vi "Check mtcdt check wifi scan.vi"(6 "VISA resource name":refnum<visa-resource-name>="COM5", 7 "Passed so far":bool, 8 "error in (no error)":errorcluster) -> (0 "error out":errorcluster, 3 "wifi mac":string, 4 "VISA Refnum out":refnum<visa-resource-name>, 5 "Passed?":bool)   [LabVIEW 2024]
panel:
  out "Response 6":string
  out "response":string
  out "Response 5":string
  out "Response 4":string
  out "Response 3":string
  out "Response 2":string
  out "Response":string
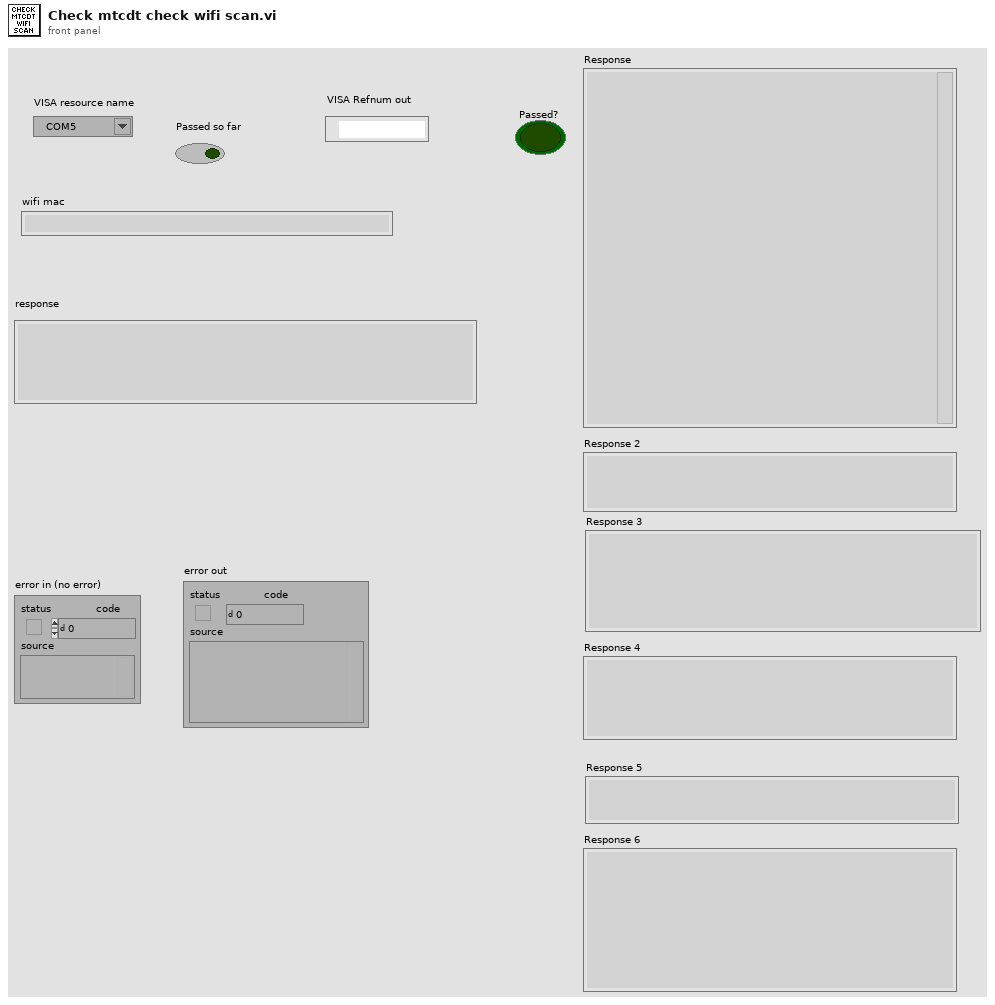
[diagram p1: front panel]
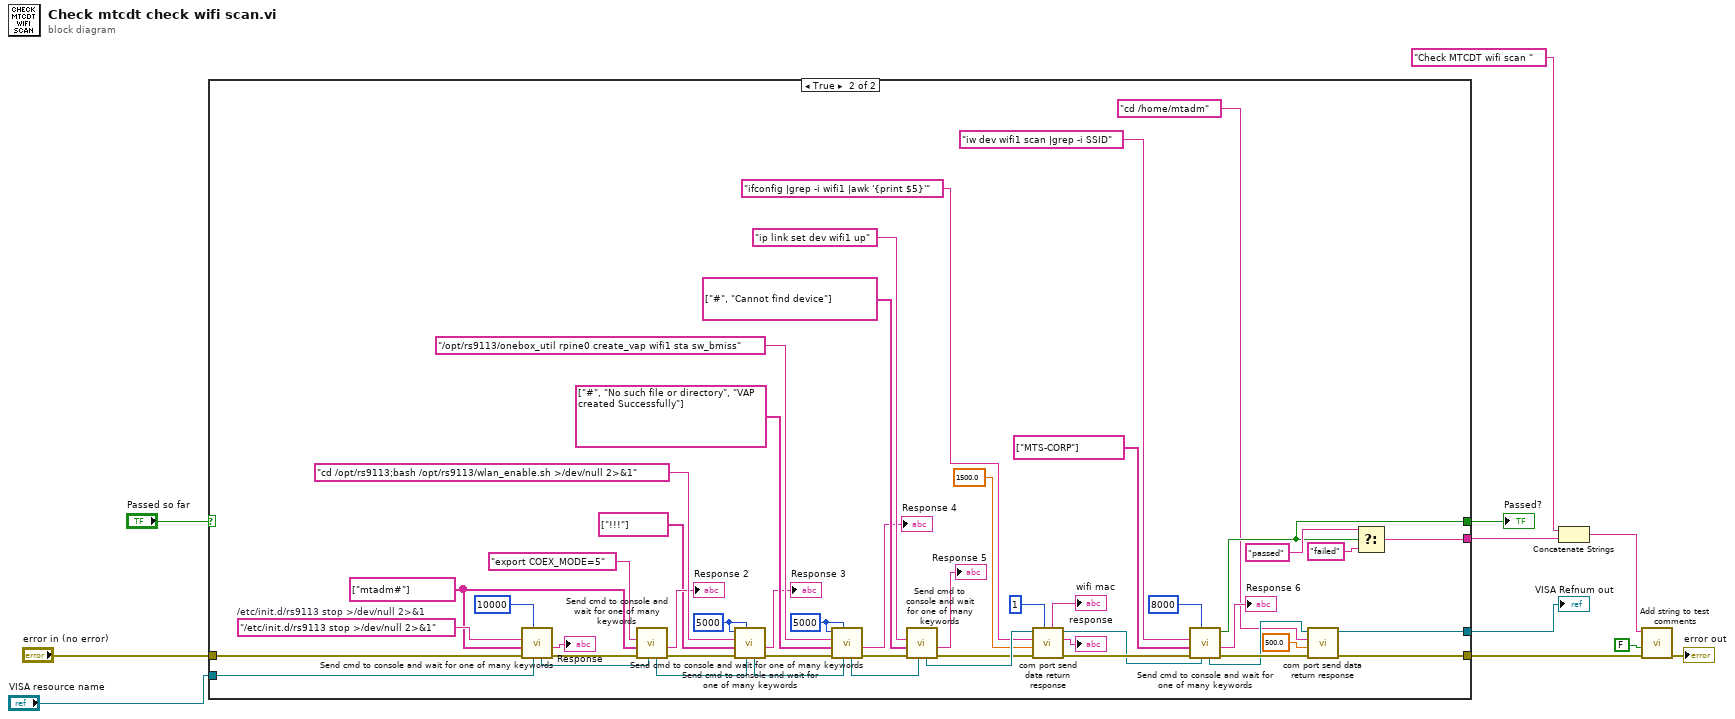
[diagram p0: block diagram]
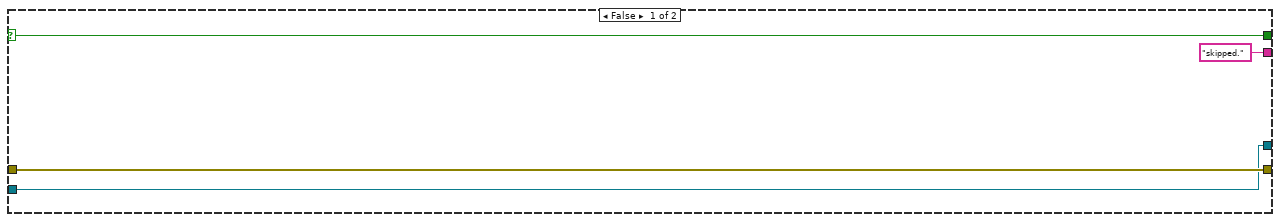
[diagram p2: hidden frame]
diagram:
  n1 = case shown="True" "Passed so far" {
    selector: "Passed so far" -> [w15 _]
    tunnel: "error in (no error)" -> [w14 w65]
    tunnel: [w14 w20] -> w2
    tunnel: "VISA resource name" -> [w13 w64]
    tunnel: [w15 w23] -> w6
    tunnel: [w13 w18] -> w4
    tunnel: ["skipped." w22] -> w1
    frame False {
    }
    frame True {
      w26 = u32 5000 ("Wait after send")
      w27 = u32 5000 ("Timeout (1000 mSecs)")
      w59 = string[] ["mtadm#"] ("Wait for keywords")
      w63 = "/etc/init.d/rs9113 stop >/dev/null 2>&1"  # /etc/init.d/rs9113 stop >/dev/null 2>&1
      n2 = call "Send cmd to console and wait for one of many keywords.vi"("VISA resource name"=w64, "Timeout (1000 mSecs)"=u32 10000, "error in (no error)"=w65, "Wait for keywords"=w59, "cmd"=w63) -> ("error out"=w60:errorcluster, "Response"=→"Response":string, "VISA Refnum out"=w62:refnum<visa-resource-name>)  [unwired: 2 in, 2 out]
      n3 = call "Send cmd to console and wait for one of many keywords.vi"("VISA resource name"=w62, "error in (no error)"=w60, "Wait for keywords"=w59, "cmd"="export COEX_MODE=5" ("write buffer")) -> ("error out"=w57:errorcluster, "Response"=→"Response 2":string, "VISA Refnum out"=w56:refnum<visa-resource-name>)  [unwired: 3 in, 2 out]
      n4 = call "Send cmd to console and wait for one of many keywords.vi"("VISA resource name"=w56, "Timeout (1000 mSecs)"=w26, "error in (no error)"=w57, "Wait for keywords"=string[] ["!!!"], "cmd"="cd /opt/rs9113;bash /opt/rs9113/wlan_enable.sh >/dev/null 2>&1" ("write buffer"), "Wait after send"=w26) -> ("error out"=w53:errorcluster, "Response"=→"Response 3":string, "VISA Refnum out"=w52:refnum<visa-resource-name>)  [unwired: 1 in, 2 out]
      n5 = call "Send cmd to console and wait for one of many keywords.vi"("VISA resource name"=w52, "Timeout (1000 mSecs)"=w27, "error in (no error)"=w53, "Wait for keywords"=string[] ["#", "No such file or directory", "VAP created Successfully"], "cmd"="/opt/rs9113/onebox_util rpine0 create_vap wifi1 sta sw_bmiss" ("write buffer"), "Wait after send"=w27) -> ("error out"=w51:errorcluster, "Response"=→"Response 4":string, "VISA Refnum out"=w50:refnum<visa-resource-name>)  [unwired: 1 in, 2 out]
      n6 = call "Send cmd to console and wait for one of many keywords.vi"("VISA resource name"=w50, "error in (no error)"=w51, "Wait for keywords"=string[] ["#", "Cannot find device"], "cmd"="ip link set dev wifi1 up" ("write buffer")) -> ("error out"=w43:errorcluster, "Response"=→"Response 5":string, "VISA Refnum out"=w47:refnum<visa-resource-name>)  [unwired: 3 in, 2 out]
      n7 = call "com port send data return response.vi"("Return line number"=u32 1, "error in (no error)"=w43, "Wait Msecs for response"=1500.0, "Send data"="ifconfig |grep -i wifi1 |awk '{print $5}'" ("write buffer"), "VISA resource name"=w47) -> ("error out"=w42:errorcluster, "response"=→"response":string, "VISA resource name out"=w40:refnum<visa-resource-name>, "Response Line"=→"wifi mac":string)  [unwired: 2 in, 1 out]
      n8 = call "Send cmd to console and wait for one of many keywords.vi"("VISA resource name"=w40, "Timeout (1000 mSecs)"=u32 8000, "error in (no error)"=w42, "Wait for keywords"=string[] ["MTS-CORP"], "cmd"="iw dev wifi1 scan |grep -i SSID" ("write buffer")) -> ("error out"=w21:errorcluster, "Response"=→"Response 6":string, "Found key?"=w23:bool, "VISA Refnum out"=w19:refnum<visa-resource-name>)  [unwired: 2 in, 1 out]
      n9 = call "com port send data return response.vi"("error in (no error)"=w21, "Wait Msecs for response"=500.0, "Send data"="cd /home/mtadm", "VISA resource name"=w19) -> ("error out"=w20:errorcluster, "VISA resource name out"=w18:refnum<visa-resource-name>)  [unwired: 3 in, 3 out]
      n10 = Select(t="passed", s=w23, f="failed") -> (s? t:f=w22:string)
    }
  }
  "Passed?" <- w6
  "VISA Refnum out" <- w4
  n11 = Concatenate Strings("Check MTCDT wifi scan " ("string"), w1) -> (w9:string)
  n12 = call "Add string to test comments.vi"("error in (no error)"=w2, "New Section (y)?"=FALSE, "Comments"=w9) -> ("error out"=→"error out":errorcluster)  [unwired: 7 in, 1 out]
